vi "Close.vi"(8 "error in":errorcluster, 11 "FileHandler in":refnum<class "FileHandler.lvclass">) -> (0 "error out":errorcluster, 3 "FileHandler out":refnum<class "FileHandler.lvclass">)   [LabVIEW 2024, in "hse-logger.lvlib" / "FileHandler.lvclass"]
doc: "Closes the log-file. This method should be called when the ``Logger`` gets closed or the handler is removed from the ``Logger``.\n\n____\nHAMPEL SOFTWARE ENGINEERING v2.2.2 (2025-01-16 15:41)"
uses:
  <vilib>/Hampel Software Engineering/HSE Logger/Handler/FileHandler/FileHandler.lvclass
  <vilib>/Hampel Software Engineering/HSE Logger/Handler/FileHandler/FileHandler.lvclass/FileHandler.ctl
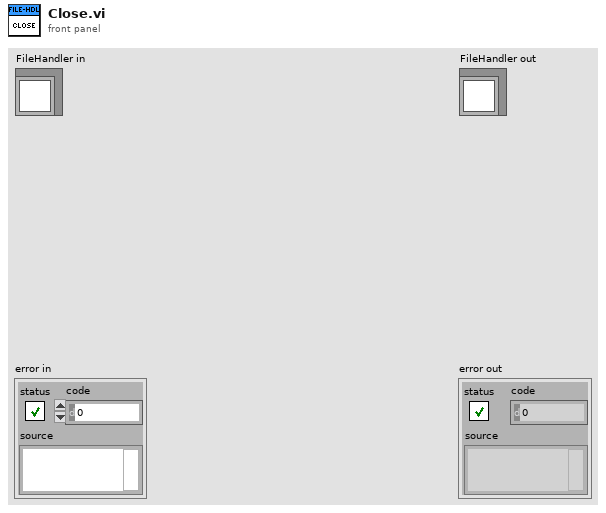
[diagram p1: front panel]
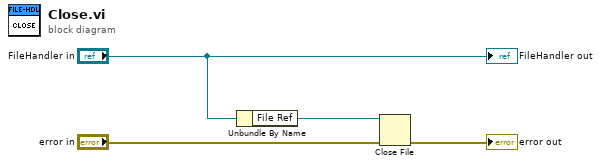
[diagram p0: block diagram]
diagram:
  n1 = Unbundle By Name("FileHandler in") -> ("File Ref"=w1:refnum<file>)
  n2 = Close File(refnum=w1, error in="error in") -> (error out=→"error out":errorcluster)  [unwired: 1 out]
  "FileHandler out" <- "FileHandler in"
